vi "GrowInfo.vi"(1 "XRef":refnum<vi>, 2 "State In":T5) -> (0 "Grow Info":T4)   [LabVIEW 2012, in "Unindex and Unbundle.xnode"]
doc: "This ability VI is used to describe your XNode's grow behavior. GrowInfo is a cluster containing the following elements:\n Min Bounds: The minimum bounds of your XNode.\n Max Bounds: The maximum bounds of your XNode.\n Vertical Increment: The vertital grow increment of your XNode. Zero is interpreted as a one pixel increment.\n Horizontal Increment: The horizontal grow increment of your XNode. Zero is interpreted as a one pixel increment.\n Maintain Aspect?: Indicates that your XNode should maintain aspect ratio.\n Oval?: Indcates that your grow lines are drawn as an oval instead of a rectangle.\n Vertical Only Resize?: Indicates that your XNode only grows vertically.\n Horizontal Only Resize?: Indicates that your XNode only grows horizontally.\n Resize None?: Indicates that your XNode can not be resized.\n\nDefault behavior: Indicate that your XNode cannot be resized.\n\nThis ability does not provide UI and OS messages are not handled.\n\nSee also: OnResize"
uses:
  Unindex and Unbundle.xnode
  State.ctl
  <vilib>/XNodeSupport/XNodeBounds.ctl
  <vilib>/XNodeSupport/XNodeInt.ctl
  <vilib>/XNodeSupport/XNodeBool.ctl
  <vilib>/XNodeSupport/NI_XNodeSupport.lvlib
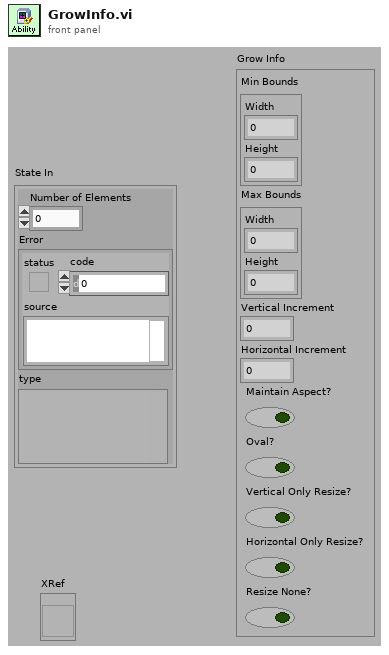
[diagram p1: front panel]
types:
  T1 = typedef "NI_XNodeSupport.lvlib/XNodeBounds.ctl" = cluster{"Width":T2, "Height":T2}
  T2 = typedef "NI_XNodeSupport.lvlib/XNodeInt.ctl" = i32
  T3 = typedef "NI_XNodeSupport.lvlib/XNodeBool.ctl" = bool
  T4 = cluster{"Min Bounds":T1, "Max Bounds":T1, "Vertical Increment":T2, "Horizontal Increment":T2, "Maintain Aspect?":T3, "Oval?":T3, "Vertical Only Resize?":T3, "Horizontal Only Resize?":T3, "Resize None?":T3}
  T5 = typedef "Unindex and Unbundle.xnode/State.ctl" = cluster{"Number of Elements":i32, "Error":errorcluster, "type":variant}
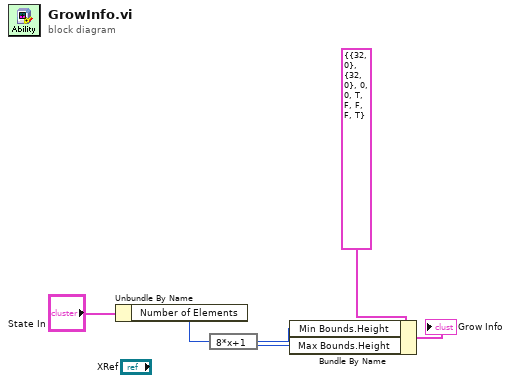
[diagram p0: block diagram]
diagram:
  n1 = Unbundle By Name("State In") -> ("Number of Elements"=w2:i32)
  n2 = expression code="8*x+1"(w2) -> (w1:i32)
  n3 = Bundle By Name(cluster=T4 {"Min Bounds"={"Width"=32, "Height"=0}, "Max Bounds"={"Width"=32, "Height"=0}, "Vertical Increment"=0, "Horizontal Increment"=0, "Maintain Aspect?"=TRUE, "Oval?"=FALSE, "Vertical Only Resize?"=FALSE, "Horizontal Only Resize?"=FALSE, "Resize None?"=TRUE} ("Grow Info"), "Min Bounds.Height"=w1, "Max Bounds.Height"=w1) -> (→"Grow Info":T4)
